vi "Stanford Research CG635 Time Capture.vi"() -> ()   [LabVIEW 2013, in "Stanford Research CG635.lvlib"]
uses:
  <instrlib>/Stanford Research CG635/Stanford Research CG635.lvlib
  <instrlib>/Stanford Research CG635/Unit Enum.ctl
panel:
  in  "CMOS High (5 V)":dbl=5.0
  in  "CMOS Low (0 V)":dbl
  in  "?":bool
  in  "Phase (0°)":i32
  in  "Unit (MHz)":T1=enum."MHz"
  out "Waveform Chart":dbl(graph)=-1.0
  in  "Frequency (10.000000 MHz)":dbl=10.0
  in  "VISA resource name":refnum<visa-resource-name>
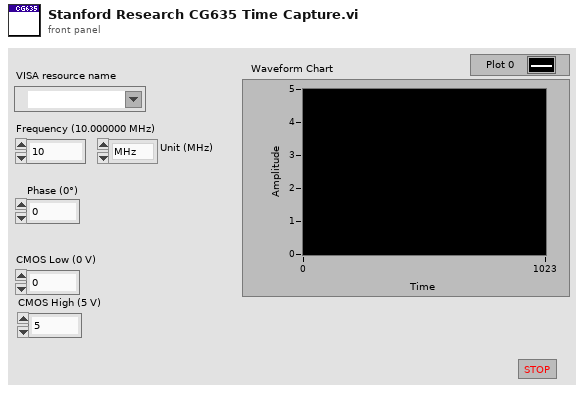
[diagram p1: front panel]
types:
  T1 = typedef "Unit Enum.ctl" = enum16{"GHz", "MHz", "kHz", "Hz"}
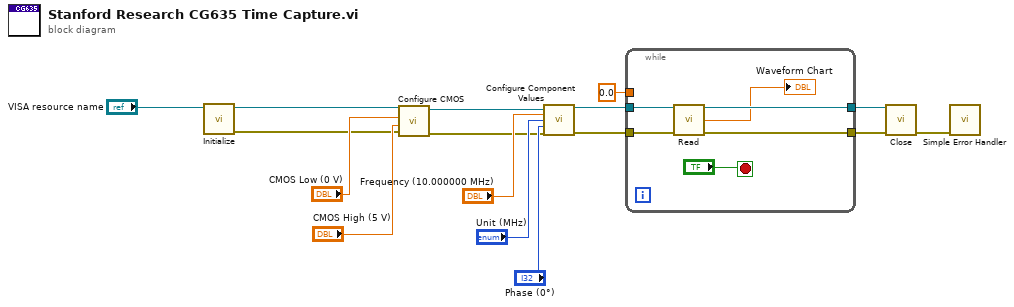
[diagram p0: block diagram]
diagram:
  n1 = call <instrlib>:"Initialize.vi"("VISA resource name"="VISA resource name") -> ("error out"=w1:errorcluster, "VISA resource name out"=w2:refnum<visa-resource-name>)  [unwired: 9 in]
  n2 = call <instrlib>:"Configure CMOS.vi"("error in (no error)"=w1, "CMOS High (5 V)"="CMOS High (5 V)", "CMOS Low (0 V)"="CMOS Low (0 V)", "VISA resource name"=w2) -> ("error out"=w3:errorcluster, "VISA resource name out"=w4:refnum<visa-resource-name>)  [unwired: 6 in]
  n3 = call <instrlib>:"Configure Component Values.vi"("VISA resource name"=w4, "Frequency (10.000000 MHz)"="Frequency (10.000000 MHz)", "Unit (MHz)"="Unit (MHz)", "Phase (0°)"="Phase (0°)", "error in (no error)"=w3) -> ("VISA resource name out"=w14:refnum<visa-resource-name>, "error out"=w13:errorcluster)  [unwired: 9 in]
  n4 = while {
    tunnel: w13 -> [w21]
    tunnel: [w19] -> w9
    tunnel: 0.0 ("double precision float") -> [_]
    tunnel: w14 -> [w22]
    tunnel: [w20] -> w10
    stop <- "?" stop-if-true
    n5 = call <instrlib>:"Read.vi"("VISA resource name"=w22, "error in (no error)"=w21) -> ("VISA resource name out"=w20:refnum<visa-resource-name>, "double precision float"=→"Waveform Chart":dbl, "error out"=w19:errorcluster)  [unwired: 11 in]
  }
  n6 = call <instrlib>:"Close.vi"("error in (no error)"=w9, "VISA resource name"=w10) -> ("error out"=w8:errorcluster)  [unwired: 9 in]
  n7 = call <vilib>:"Simple Error Handler.vi"("error in (no error)"=w8) -> ()  [unwired: 4 in, 5 out]
